vi "Draw Single Icon.vi"(8 "error in (no error)":errorcluster, 10 "Icon Index":i32, 11 "Toolbar Control in":refnum<class "Toolbar Control.lvclass">) -> (0 "error out":errorcluster, 3 "Toolbar Control out":refnum<class "Toolbar Control.lvclass">)   [LabVIEW 2011, in "Toolbar Control.lvclass"]
doc: "This VI will draw a single icon form the <B>Icon Index</B> selection.\n\n-------------\nDeveloped by Brian Hoover (hooovahh)"
uses:
  Toolbar Control.lvclass
  Toolbar Control.lvclass/Toolbar Control.ctl
  <vilib>/Utility/miscctls.llb/LVBoundsTypeDef.ctl
  Controls/Mouse State.ctl
  Non Class Utilities/Convert to 32Bit Image.vi
  <vilib>/Utility/colorconv.llb/Color to RGB.vi
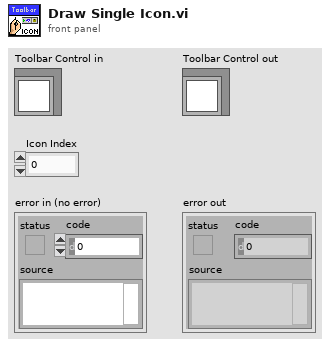
[diagram p1: front panel]
types:
  T1 = typedef "Mouse State.ctl" = enum8{"Normal", "Mouse Over", "Mouse Down"}
  T2 = typedef "LVBoundsTypeDef.ctl" = cluster{"Width":u32, "Height":u32}
  T3 = enum16{"User-specified Font", "Application Font", "System Font", "Dialog Font"}
  T4 = typedef "LVRectTypeDef.ctl" = cluster{"Left":i16, "Top":i16, "Right":i16, "Bottom":i16}
  T5 = typedef "Toolbar Control.lvclass/Icon Data.ctl" = cluster{"Original Image Path":path, "Original Image Data":T6, "Scaled Icon":picture, "Button Name":string, "Button State":T7, "Icon Type":T8}
  T6 = typedef "imagedata.ctl" = cluster{"image type":i32, "image depth":i32, "image":u8[], "mask":u8[], "colors":u32[], "Rectangle":cluster{"left":i16, "top":i16, "right":i16, "bottom":i16}}
  T7 = typedef "Toolbar Control.lvclass/Button State.ctl" = enum8{"Enabled", "Disabled", "Disabled and Grayed Out"}
  T8 = typedef "Icon Type.ctl" = enum16{"Normal Icon", "Separator Icon", "More Options"}
  T9 = cluster{"left":i16, "top":i16, "right":i16, "bottom":i16}
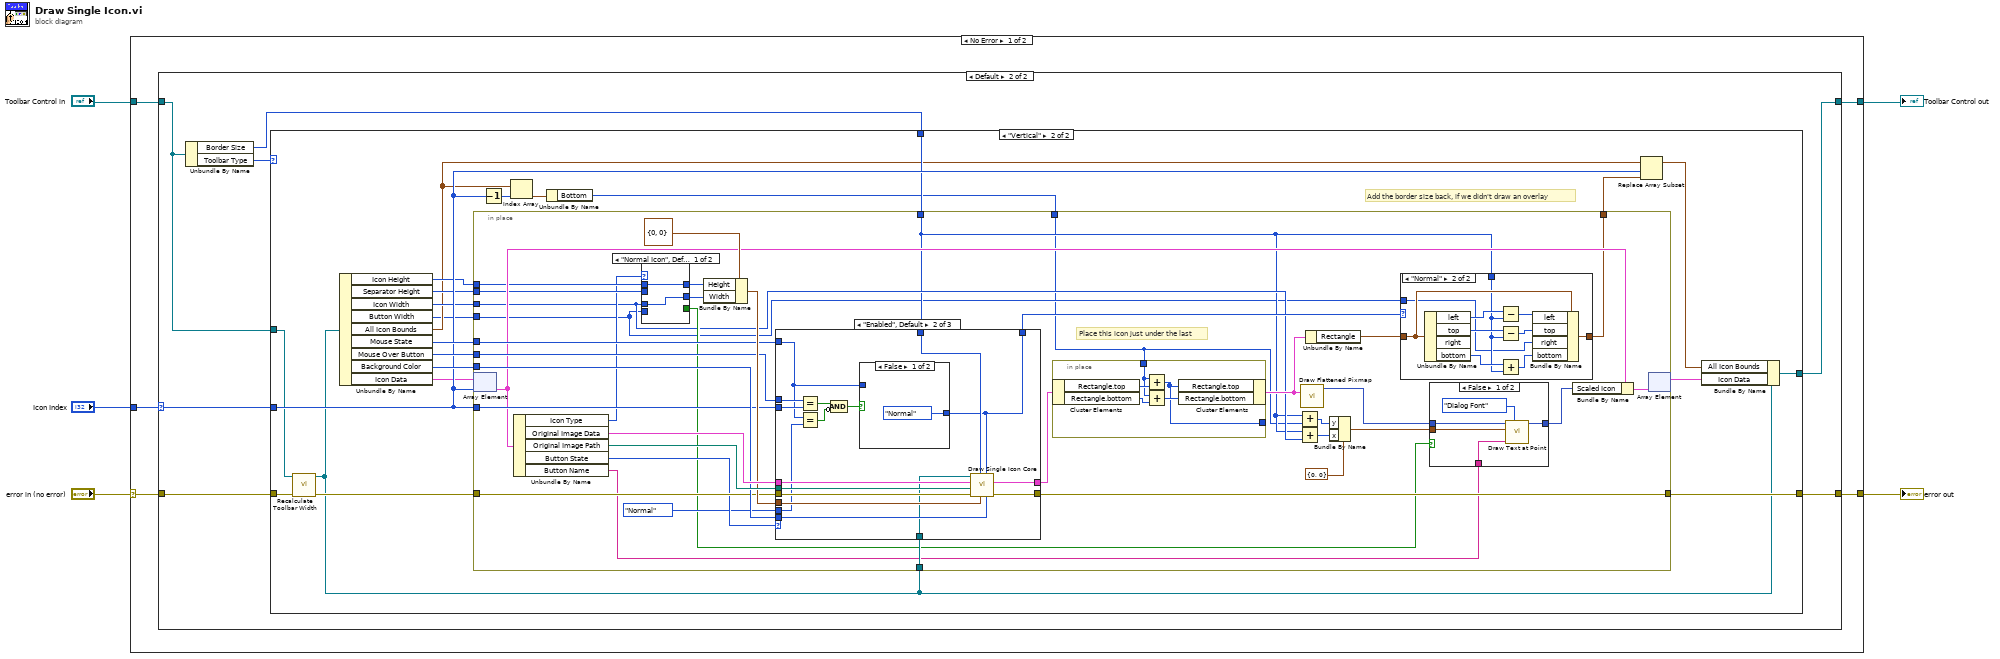
[diagram p0: block diagram]
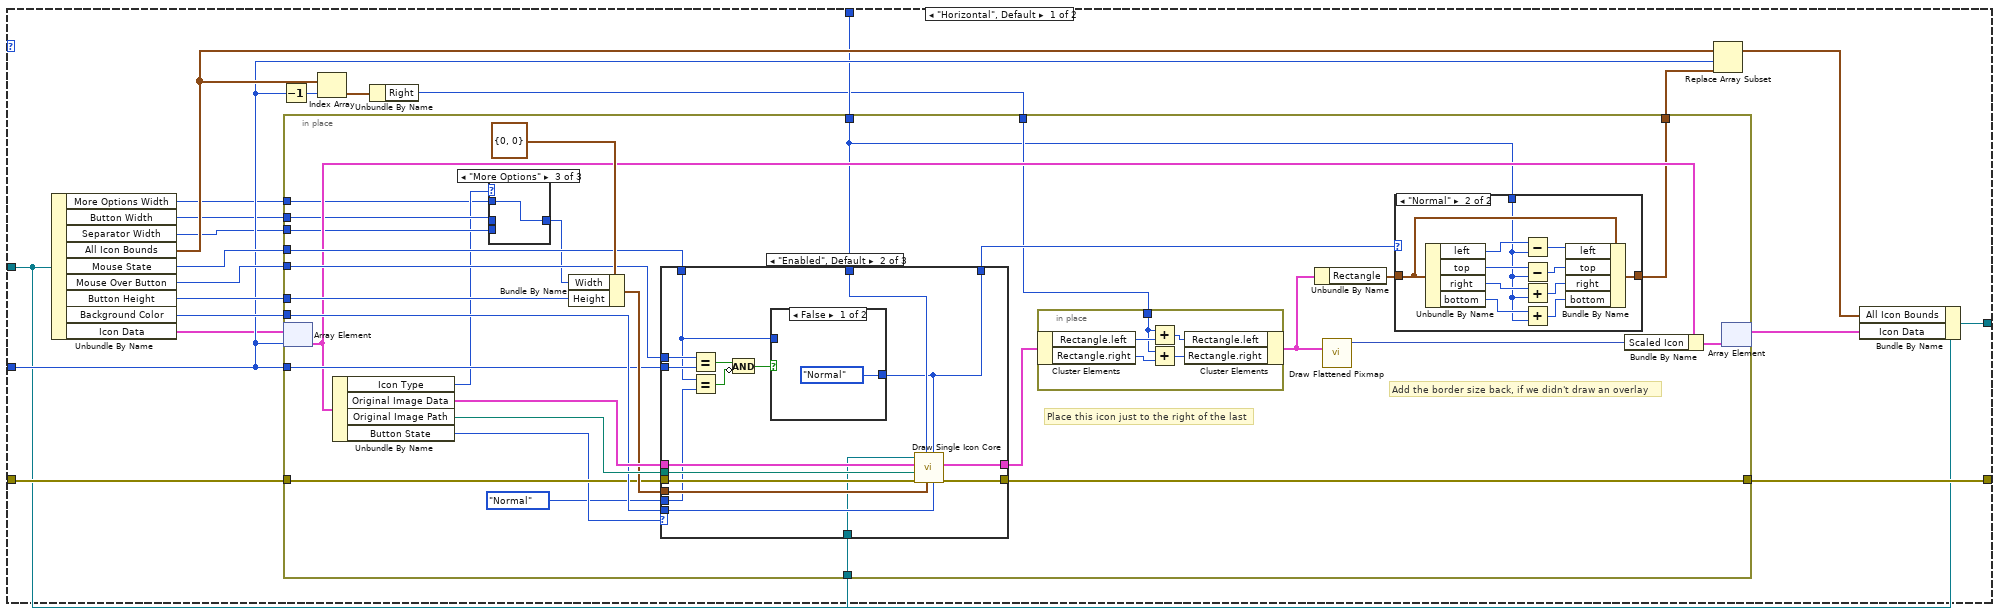
[diagram p3: hidden frame]
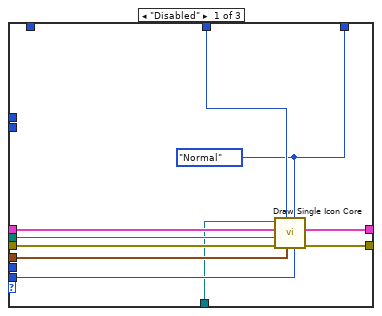
[diagram p7: hidden frame]
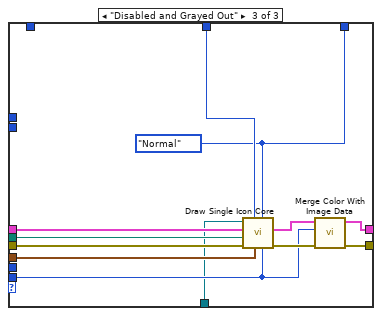
[diagram p9: hidden frame]
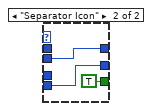
[diagram p11: hidden frame]
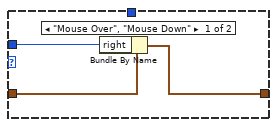
[diagram p12: hidden frame]
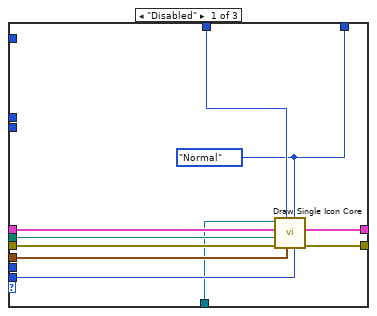
[diagram p13: hidden frame]
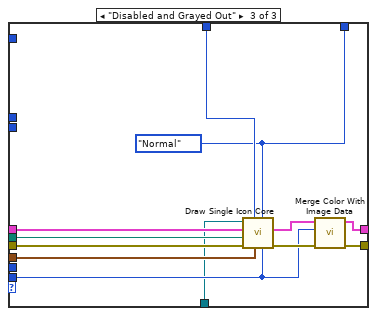
[diagram p15: hidden frame]
diagram:
  n1 = case shown="No Error" "error in (no error)" {
    selector: "error in (no error)" -> [w10 w262]
    tunnel: [w9 w262] -> w4
    tunnel: [w8 w261] -> w2
    tunnel: "Toolbar Control in" -> [w6 w261]
    tunnel: "Icon Index" -> [w7 _]
    frame No Error {
      n2 = case shown="Default" w7 {
        selector: w7 -> [_ w16]
        tunnel: w6 -> [w12 w14]
        tunnel: w10 -> [w11 w19]
        tunnel: [w11 w18] -> w9
        tunnel: [w12 w17] -> w8
        frame -1 {
        }
        frame Default {
          n3 = Unbundle By Name(w14) -> ("Border Size"=w13:i16, "Toolbar Type"=w15:enum16{"Horizontal", "Vertical"})
          n4 = case shown="\"Vertical\"" w15 {
            tunnel: w19 -> [w38 w134]
            tunnel: [w37 w152] -> w18
            tunnel: [w34 w149] -> w17
            tunnel: w16 -> [w31 w147]
            tunnel: w13 -> [w26 w143]
            tunnel: w14 -> [w20 w132]
            frame "Horizontal", Default {
              n5 = Unbundle By Name(w20) -> ("More Options Width"=w27:i32, "Button Width"=w29:i32, "Separator Width"=w28:i32, "All Icon Bounds"=w32:T4[], "Mouse State"=w35:T1, "Mouse Over Button"=w36:i32, "Button Height"=w39:i32, "Background Color"=w40:u32, "Icon Data"=w25:T5[])
              n6 = Decrement(x=w31) -> (x-1=w24:i32)
              n7 = Index Array(array=w32, index=w24) -> (element=w23:T4)
              n8 = Unbundle By Name(w23) -> ("Right"=w22:i16)
              n9 = in-place {
                in-place-border: w40 -> [w67]
                in-place-border: w39 -> [w64]
                in-place-border: w38 -> [w63]
                in-place-border: [w62] -> w37
                in-place-border: w31 -> [w60]
                in-place-border: w36 -> [w59]
                in-place-border: w35 -> [w58]
                in-place-border: w20 -> [w51]
                in-place-border: w22 -> [w47]
                in-place-border: [w49] -> w21
                in-place-border: w29 -> [w46]
                in-place-border: w28 -> [w45]
                in-place-border: w27 -> [w42]
                in-place-border: w26 -> [w41]
                # "Add the border size back, if we didn't draw an overlay"
                # "Place this icon just to the right of the last"
                n10 = in-place-array #1(w25, w31) -> (w55:T5)
                n11 = Unbundle By Name(w55) -> ("Icon Type"=w43:T8, "Original Image Data"=w69:T6, "Original Image Path"=w68:path, "Button State"=w61:T7)
                n12 = case shown="\"More Options\"" w43 {
                  tunnel: w46 -> [w70 _ _]
                  tunnel: w45 -> [_ w71 _]
                  tunnel: [w70 w71 w72] -> w44
                  tunnel: w42 -> [_ _ w72]
                  frame "Normal Icon", Default {
                  }
                  frame "Separator Icon" {
                  }
                  frame "More Options" {
                  }
                }
                n13 = Bundle By Name(cluster=T2 {"Width"=0, "Height"=0} ("Icon Size"), "Width"=w44, "Height"=w64) -> (w65:T2)
                n14 = case shown="\"Enabled\", Default" w61 {
                  tunnel: w69 -> [w99 w116 w130]
                  tunnel: w68 -> [w98 w115 w129]
                  tunnel: w67 -> [w93 w104 w122]
                  tunnel: w65 -> [w97 w114 w128]
                  tunnel: w63 -> [w96 w113 w127]
                  tunnel: [w95 w112 w125] -> w62
                  tunnel: w60 -> [_ w108 _]
                  tunnel: w59 -> [_ w107 _]
                  tunnel: w58 -> [_ w105 _]
                  tunnel: Mouse_State."Normal" ("Mouse State") -> [_ w106 _]
                  tunnel: [w94 w103 w124] -> w53
                  tunnel: w51 -> [w92 w102 w121]
                  tunnel: w41 -> [w91 w101 w120]
                  tunnel: [w90 w100 w119] -> w48
                  frame "Disabled" {
                    w90 = Mouse_State."Normal" ("Mouse State")
                    n15 = call "Draw Single Icon Core.vi"("Background Color"=w93, "Mouse State"=w90, "Icon Size"=w97, "Border Size"=w91, "error in (no error)"=w96, "Image Path"=w98, "Image Data"=w99, "Toolbar Control in"=w92) -> ("error out"=w95:errorcluster, "Icon Image Out"=w94:T6)  [unwired: 1 in, 1 out]
                  }
                  frame "Enabled", Default {
                    n16 = Equal?(x=w107, y=w108) -> (x = y?=w111:bool)
                    n17 = Equal?(x=w105, y=w106) -> (x = y?=w110:bool)
                    n18 = Compound Arithmetic op=AND(w111, invert w110) -> (w109:bool)
                    n19 = case shown="False" w109 {
                      tunnel: [Mouse_State."Normal" ("Mouse State") w118] -> w100
                      tunnel: w105 -> [_ w118]
                      frame False {
                      }
                      frame True {
                      }
                    }
                    n20 = call "Draw Single Icon Core.vi"("Background Color"=w104, "Mouse State"=w100, "Icon Size"=w114, "Border Size"=w101, "error in (no error)"=w113, "Image Path"=w115, "Image Data"=w116, "Toolbar Control in"=w102) -> ("error out"=w112:errorcluster, "Icon Image Out"=w103:T6)  [unwired: 1 in, 1 out]
                  }
                  frame "Disabled and Grayed Out" {
                    w119 = Mouse_State."Normal" ("Mouse State")
                    n21 = call "Draw Single Icon Core.vi"("Background Color"=w122, "Mouse State"=w119, "Icon Size"=w128, "Border Size"=w120, "error in (no error)"=w127, "Image Path"=w129, "Image Data"=w130, "Toolbar Control in"=w121) -> ("error out"=w126:errorcluster, "Icon Image Out"=w123:T6)  [unwired: 1 in, 1 out]
                    n22 = call "Merge Color With Image Data.vi"("error in (no error)"=w126, "Color"=w122, "Image Data in"=w123) -> ("error out"=w125:errorcluster, "Image Data out"=w124:T6)  [unwired: 7 in]
                  }
                }
                n23 = in-place {
                  in-place-border: w47 -> [w73]
                  n24 = in-place-cluster #2(w53) -> ("Rectangle.left"=w77:i16, "Rectangle.right"=w76:i16)
                  n25 = Add(x=w73, y=w77) -> (x+y=w75:i16)
                  n26 = Add(x=w73, y=w76) -> (x+y=w74:i16)
                  n27 = in-place-cluster #2("Rectangle.left"=w75, "Rectangle.right"=w74) -> (w52:T6)
                }
                n28 = Unbundle By Name(w52) -> ("Rectangle"=w50:T9)
                n29 = call <vilib>:"Draw Flattened Pixmap.vi"("image data"=w52) -> ("new picture"=w56:picture)  [unwired: 8 in]
                n30 = case shown="\"Normal\"" w48 {
                  tunnel: w50 -> [w78 w89]
                  tunnel: [w78 w88] -> w49
                  tunnel: w41 -> [_ w81]
                  frame "Mouse Over", "Mouse Down" {
                  }
                  frame "Normal" {
                    n31 = Unbundle By Name(w89) -> ("left"=w87:i16, "top"=w86:i16, "right"=w83:i16, "bottom"=w82:i16)
                    n32 = Subtract(x=w87, y=w81) -> (x-y=w85:i16)
                    n33 = Subtract(x=w86, y=w81) -> (x-y=w84:i16)
                    n34 = Add(x=w83, y=w81) -> (x+y=w80:i16)
                    n35 = Add(x=w82, y=w81) -> (x+y=w79:i16)
                    n36 = Bundle By Name(cluster=w89, "left"=w85, "top"=w84, "right"=w80, "bottom"=w79) -> (w88:T9)
                  }
                }
                n37 = Bundle By Name(cluster=w55, "Scaled Icon"=w56) -> (w54:T5)
                n38 = in-place-array #1(w54) -> (w33:T5[])  [unwired: 1 out]
              }
              n39 = Replace Array Subset(array=w32, new element=w21, index=w31) -> (w30:T4[])
              n40 = Bundle By Name(cluster=w20, "All Icon Bounds"=w30, "Icon Data"=w33) -> (w34:refnum<class "Toolbar Control.lvclass">)
            }
            frame "Vertical" {
              # "Add the border size back, if we didn't draw an overlay"
              n41 = call "Recalculate Toolbar Width.vi"("error in (no error)"=w134, "Toolbar Control in"=w132) -> ("error out"=w133:errorcluster, "Toolbar Control out"=w131:refnum<class "Toolbar Control.lvclass">)  [unwired: 8 in]
              n42 = Unbundle By Name(w131) -> ("Icon Height"=w145:i32, "Separator Height"=w144:i32, "Icon Width"=w137:i32, "Button Width"=w135:i32, "All Icon Bounds"=w136:T4[], "Mouse State"=w150:T1, "Mouse Over Button"=w151:i32, "Background Color"=w153:u32, "Icon Data"=w142:T5[])
              n43 = Decrement(x=w147) -> (x-1=w141:i32)
              n44 = Index Array(array=w136, index=w141) -> (element=w140:T4)
              n45 = Unbundle By Name(w140) -> ("Bottom"=w139:i16)
              n46 = in-place {
                in-place-border: w153 -> [w188]
                in-place-border: w133 -> [w185]
                in-place-border: [w184] -> w152
                in-place-border: w147 -> [w182]
                in-place-border: w151 -> [w181]
                in-place-border: w150 -> [w180]
                in-place-border: w131 -> [w174]
                in-place-border: w139 -> [w154]
                in-place-border: [w172] -> w138
                in-place-border: w145 -> [w170]
                in-place-border: w144 -> [w169]
                in-place-border: w143 -> [w156]
                in-place-border: w137 -> [w157]
                in-place-border: w135 -> [w155]
                # "Place this icon just under the last"
                n47 = in-place-array #3(w142, w147) -> (w178:T5)
                n48 = Unbundle By Name(w178) -> ("Icon Type"=w167:T8, "Original Image Data"=w190:T6, "Original Image Path"=w189:path, "Button State"=w183:T7, "Button Name"=w163:string)
                n49 = case shown="\"Normal Icon\", Default" w167 {
                  tunnel: w170 -> [w198 _]
                  tunnel: w169 -> [_ w201]
                  tunnel: [w198 w201] -> w168
                  tunnel: w157 -> [w197 _]
                  tunnel: w155 -> [_ w200]
                  tunnel: [w197 w200] -> w166
                  tunnel: [_ TRUE] -> w159
                  frame "Normal Icon", Default {
                  }
                  frame "Separator Icon" {
                  }
                }
                n50 = Bundle By Name(cluster=T2 {"Width"=0, "Height"=0} ("Icon Size"), "Height"=w168, "Width"=w166) -> (w186:T2)
                n51 = case shown="\"Enabled\", Default" w183 {
                  tunnel: w190 -> [w229 w246 w260]
                  tunnel: w189 -> [w228 w245 w259]
                  tunnel: w188 -> [w223 w234 w252]
                  tunnel: w186 -> [w227 w244 w258]
                  tunnel: w185 -> [w226 w243 w257]
                  tunnel: [w225 w242 w255] -> w184
                  tunnel: w182 -> [_ w238 _]
                  tunnel: w181 -> [_ w237 _]
                  tunnel: w180 -> [_ w235 _]
                  tunnel: Mouse_State."Normal" ("Mouse State") -> [_ w236 _]
                  tunnel: [w224 w233 w254] -> w176
                  tunnel: w174 -> [w222 w232 w251]
                  tunnel: w156 -> [w221 w231 w250]
                  tunnel: [w220 w230 w249] -> w171
                  frame "Disabled" {
                    w220 = Mouse_State."Normal" ("Mouse State")
                    n52 = call "Draw Single Icon Core.vi"("Background Color"=w223, "Mouse State"=w220, "Icon Size"=w227, "Border Size"=w221, "error in (no error)"=w226, "Image Path"=w228, "Image Data"=w229, "Toolbar Control in"=w222) -> ("error out"=w225:errorcluster, "Icon Image Out"=w224:T6)  [unwired: 1 in, 1 out]
                  }
                  frame "Enabled", Default {
                    n53 = Equal?(x=w237, y=w238) -> (x = y?=w241:bool)
                    n54 = Equal?(x=w235, y=w236) -> (x = y?=w240:bool)
                    n55 = Compound Arithmetic op=AND(w241, invert w240) -> (w239:bool)
                    n56 = case shown="False" w239 {
                      tunnel: [Mouse_State."Normal" ("Mouse State") w248] -> w230
                      tunnel: w235 -> [_ w248]
                      frame False {
                      }
                      frame True {
                      }
                    }
                    n57 = call "Draw Single Icon Core.vi"("Background Color"=w234, "Mouse State"=w230, "Icon Size"=w244, "Border Size"=w231, "error in (no error)"=w243, "Image Path"=w245, "Image Data"=w246, "Toolbar Control in"=w232) -> ("error out"=w242:errorcluster, "Icon Image Out"=w233:T6)  [unwired: 1 in, 1 out]
                  }
                  frame "Disabled and Grayed Out" {
                    w249 = Mouse_State."Normal" ("Mouse State")
                    n58 = call "Draw Single Icon Core.vi"("Background Color"=w252, "Mouse State"=w249, "Icon Size"=w258, "Border Size"=w250, "error in (no error)"=w257, "Image Path"=w259, "Image Data"=w260, "Toolbar Control in"=w251) -> ("error out"=w256:errorcluster, "Icon Image Out"=w253:T6)  [unwired: 1 in, 1 out]
                    n59 = call "Merge Color With Image Data.vi"("error in (no error)"=w256, "Color"=w252, "Image Data in"=w253) -> ("error out"=w255:errorcluster, "Image Data out"=w254:T6)  [unwired: 7 in]
                  }
                }
                n60 = in-place {
                  in-place-border: w154 -> [w203]
                  in-place-border: [w202] -> _
                  n61 = in-place-cluster #4(w176) -> ("Rectangle.top"=w206:i16, "Rectangle.bottom"=w205:i16)
                  n62 = Add(x=w203, y=w206) -> (x+y=w202:i16)
                  n63 = Add(x=w203, y=w205) -> (x+y=w204:i16)
                  n64 = in-place-cluster #4("Rectangle.top"=w202, "Rectangle.bottom"=w204) -> (w175:T6)
                }
                n65 = Add(x=w156, y=w154) -> (x+y=w158:i16)
                n66 = Add(x=w156, y=w157) -> (x+y=w160:i32)
                n67 = call <vilib>:"Draw Flattened Pixmap.vi"("image data"=w175) -> ("new picture"=w165:picture)  [unwired: 8 in]
                n68 = Unbundle By Name(w175) -> ("Rectangle"=w173:T9)
                n69 = Bundle By Name(cluster=cluster{"x":i16, "y":i16} {"x"=0, "y"=0} ("origin"), "y"=w158, "x"=w160) -> (w161:cluster{"x":i16, "y":i16})
                n70 = case shown="\"Normal\"" w171 {
                  tunnel: w173 -> [w209 w219]
                  tunnel: [w208 w218] -> w172
                  tunnel: w156 -> [_ w212]
                  tunnel: w155 -> [w207 w210]
                  frame "Mouse Over", "Mouse Down" {
                    n71 = Bundle By Name(cluster=w209, "right"=w207) -> (w208:T9)
                  }
                  frame "Normal" {
                    n72 = Unbundle By Name(w219) -> ("left"=w217:i16, "top"=w216:i16, "bottom"=w213:i16)  [unwired: 1 out]
                    n73 = Subtract(x=w217, y=w212) -> (x-y=w215:i16)
                    n74 = Subtract(x=w216, y=w212) -> (x-y=w214:i16)
                    n75 = Add(x=w213, y=w212) -> (x+y=w211:i16)
                    n76 = Bundle By Name(cluster=w219, "left"=w215, "top"=w214, "right"=w210, "bottom"=w211) -> (w218:T9)
                  }
                }
                n77 = case shown="False" w159 {
                  tunnel: w165 -> [w195 w196]
                  tunnel: [w194 w196] -> w164
                  tunnel: w163 -> [w192 _]
                  tunnel: w161 -> [w191 _]
                  frame False {
                    n78 = call <vilib>:"Draw Text at Point.vi"("desired font(Application)"=T3."Dialog Font", "text"=w192, "origin"=w191, "picture"=w195) -> ("new picture"=w194:picture)  [unwired: 6 in, 1 out]
                  }
                  frame True {
                  }
                }
                n79 = Bundle By Name(cluster=w178, "Scaled Icon"=w164) -> (w177:T5)
                n80 = in-place-array #3(w177) -> (w148:T5[])  [unwired: 1 out]
              }
              n81 = Replace Array Subset(array=w136, new element=w138, index=w147) -> (w146:T4[])
              n82 = Bundle By Name(cluster=w131, "All Icon Bounds"=w146, "Icon Data"=w148) -> (w149:refnum<class "Toolbar Control.lvclass">)
            }
          }
        }
      }
    }
    frame Error {
    }
  }
  "error out" <- w4
  "Toolbar Control out" <- w2
